vi "Counter_Divideby4.vi"() -> ()   [LabVIEW 2012]
uses:
  <vilib>/Waveform/DTblOps.llb/DTbl Boolean Array to Digital.vi
panel:
  out "Digital Waveform Graph":digitaldata(graph)
  in  "millisecond multiple":u32
  out "Q4":bool
  out "Q3":bool
  out "Q1":bool
  out "Q2":bool
  in  "Slices":u32
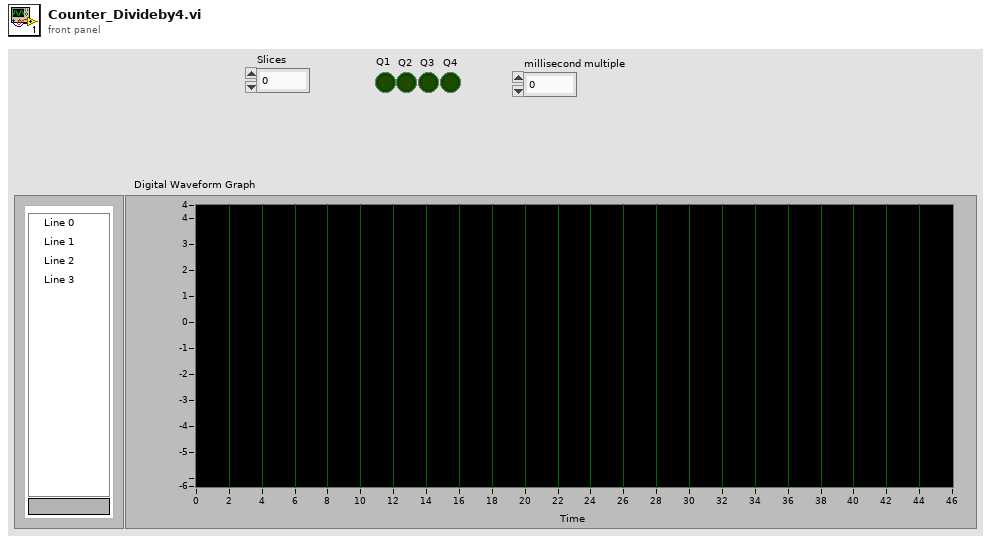
[diagram p1: front panel]
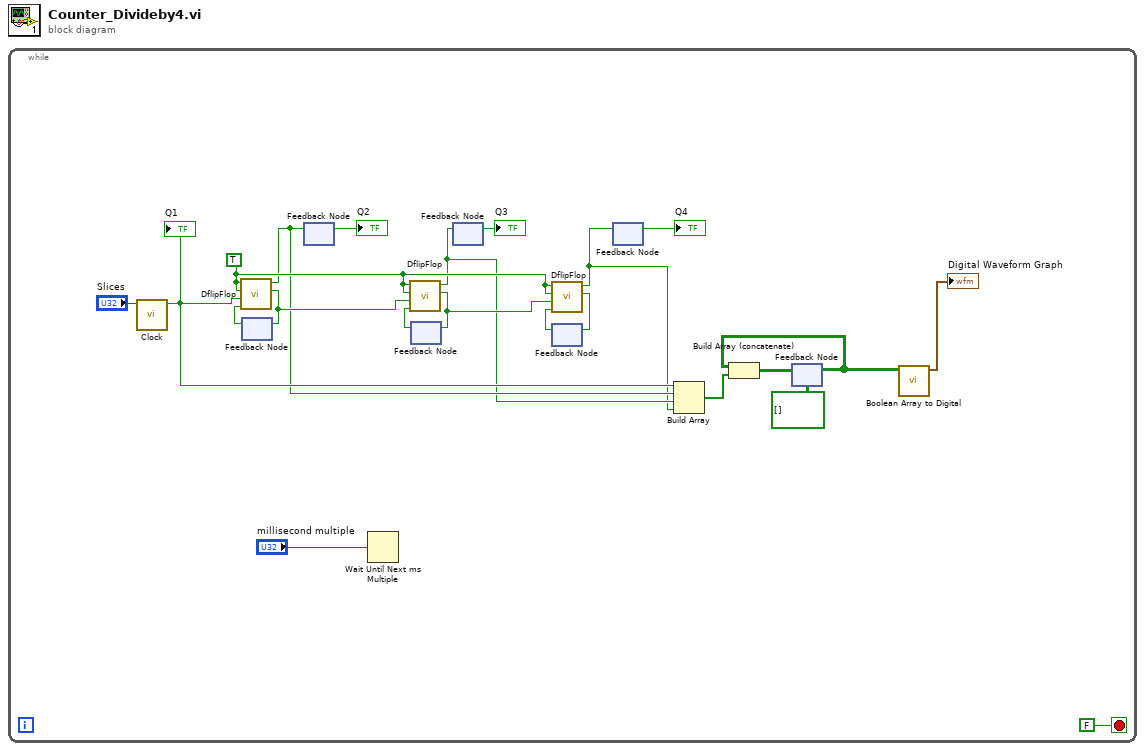
[diagram p0: block diagram]
diagram:
  n1 = while {
    stop <- FALSE stop-if-true
    w21 = TRUE ("Set")
    n2 = call "Clock.vi"("Slices"="Slices") -> ("Clk"=w9:bool)  [unwired: 10 in]
    "Q1" <- w9
    n3 = feedback #1() -> (w19:bool)  [unwired: 1 in]
    n4 = call "DflipFlop.vi"("D"=w19, "Clock"=w9, "Reset"=w21, "Set"=w21) -> ("/Q\\"=w15:bool, "Q"=w3:bool)  [unwired: 6 in]
    n5 = feedback-in #1(w15) -> ()
    n6 = feedback-in #2(w3) -> ()
    n7 = feedback #2() -> (→"Q2":bool)  [unwired: 1 in]
    n8 = Wait Until Next ms Multiple(millisecond multiple="millisecond multiple") -> ()  [unwired: 1 out]
    n9 = feedback #3() -> (w18:bool)  [unwired: 1 in]
    n10 = call "DflipFlop.vi"("D"=w18, "Clock"=w15, "Reset"=w21, "Set"=w21) -> ("/Q\\"=w14:bool, "Q"=w2:bool)  [unwired: 6 in]
    n11 = feedback-in #3(w14) -> ()
    n12 = feedback #4() -> (→"Q3":bool)  [unwired: 1 in]
    n13 = feedback-in #4(w2) -> ()
    n14 = feedback #5() -> (w16:bool)  [unwired: 1 in]
    n15 = call "DflipFlop.vi"("D"=w16, "Clock"=w14, "Reset"=w21, "Set"=w21) -> ("/Q\\"=w17:bool, "Q"=w1:bool)  [unwired: 6 in]
    n16 = feedback-in #5(w17) -> ()
    n17 = feedback #6() -> (→"Q4":bool)  [unwired: 1 in]
    n18 = feedback-in #6(w1) -> ()
    n19 = Build Array(w9, w3, w2, w1) -> (w5:bool[])
    n20 = feedback #7(bool[][] []) -> (w10:bool[][])
    n21 = Build Array (concatenate)(w10, w5) -> (w12:bool[][])
    n22 = feedback-in #7(w12) -> ()
    n23 = call-poly <vilib>:"Boolean Array to Digital.vi"("boolean array"=w10) -> ("digital data"=→"Digital Waveform Graph":digitaldata)  [unwired: 9 in, 1 out]
  }
